vi "Change Sub Panel VI.vi"(8 "error in (no error)":errorcluster, 11 "TestBench in":refnum<class "TestBench.lvclass">) -> (0 "error out":errorcluster, 3 "TestBench out":refnum<class "TestBench.lvclass">)   [LabVIEW 2019, in "TestBench.lvlib" / "TestBench.lvclass"]
uses:
  TestBench.lvclass
  TestBench.lvclass/TestBench.ctl
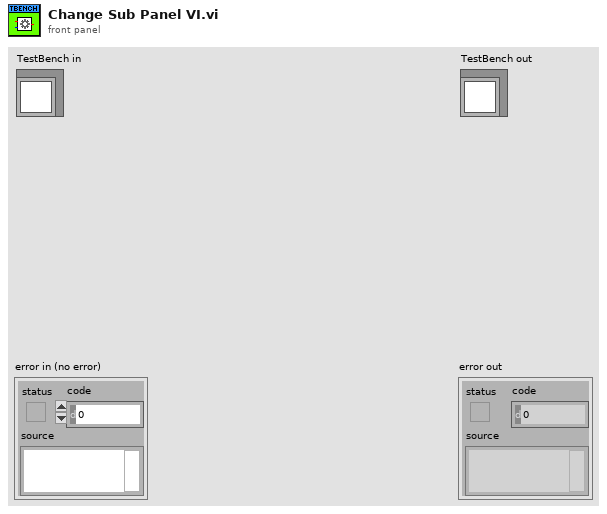
[diagram p1: front panel]
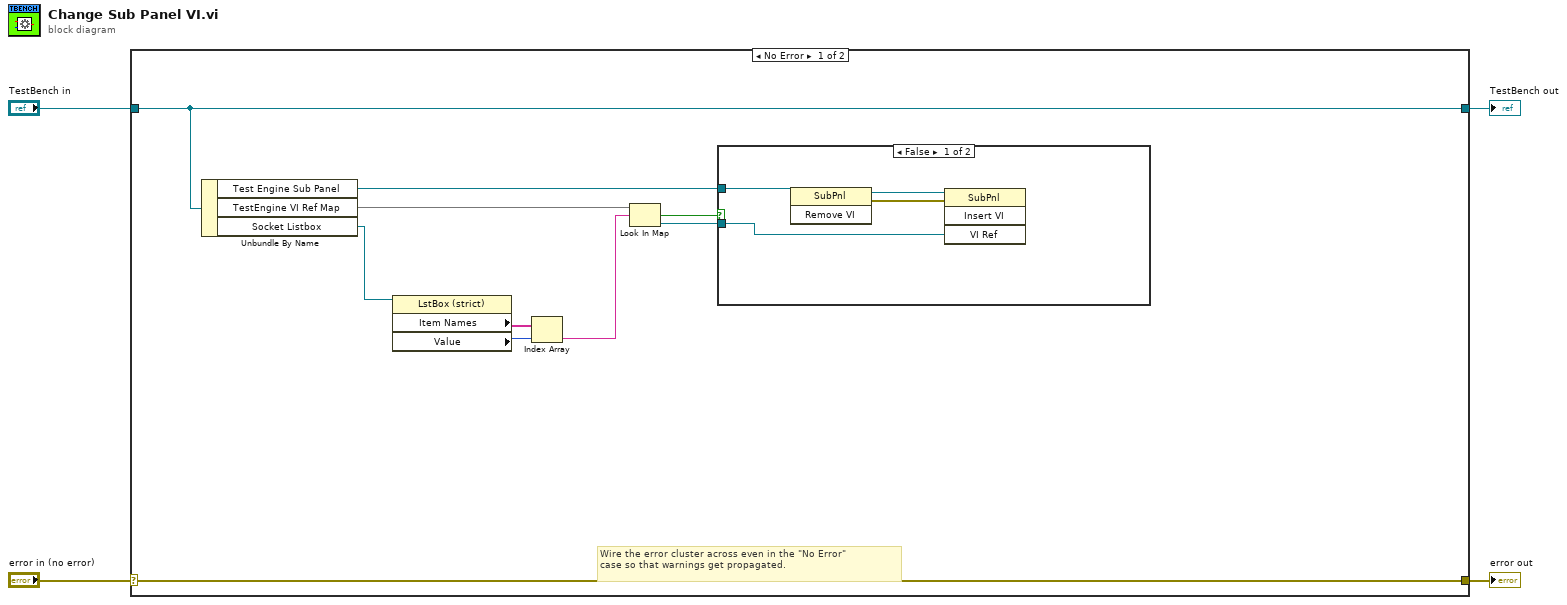
[diagram p0: block diagram]
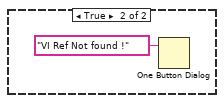
[diagram p2: hidden frame]
diagram:
  n1 = case shown="No Error" "error in (no error)" {
    selector: "error in (no error)" -> [w14 w21]
    tunnel: [w14 w21] -> w3
    tunnel: [w13 w20] -> w1
    tunnel: "TestBench in" -> [w13 w20]
    frame No Error {
      # "Wire the error cluster across even in the \"No Error\"\ncase so that warnings get propagated."
      n2 = Unbundle By Name(w13) -> ("Test Engine Sub Panel"=w12:refnum<vi>, "TestEngine VI Ref Map"=w11:map{string, refnum<vi>}, "Socket Listbox"=w10:refnum<vi>)
      n3 = property class="LstBox (strict)"(reference=w10) -> ("Item Names"=w9:string[], "Value"=w8:i32)  [unwired: 1 in, 2 out]
      n4 = Index Array(array=w9, index=w8) -> (element=w7:string)
      n5 = Look In Map(map=w11, key=w7) -> (key not found?=w5:bool, value=w6:refnum<vi>)  [unwired: 1 in]
      n6 = case shown="False" w5 {
        tunnel: w12 -> [w17 _]
        tunnel: w6 -> [w16 _]
        frame False {
          n7 = invoke class="SubPnl" method="Remove VI"(reference=w17) -> (reference out=w15:refnum<vi>, error out=w18:errorcluster)  [unwired: 2 in, 1 out]
          n8 = invoke class="SubPnl" method="Insert VI"(reference=w15, error in=w18, "VI Ref"=w16) -> ()  [unwired: 1 in, 4 out]
        }
        frame True {
          n9 = One Button Dialog(message="VI Ref Not found !") -> ()  [unwired: 1 in, 1 out]
        }
      }
    }
    frame Error {
    }
  }
  "error out" <- w3
  "TestBench out" <- w1
